vi "Initialize.vi"(8 "error in (no error)":errorcluster caption="错误输入（无错误）", 11 "虚拟 输入":refnum<class "虚拟.lvclass">) -> (0 "error out":errorcluster caption="错误输出", 3 "虚拟 输出":refnum<class "虚拟.lvclass">)   [LabVIEW 2020, in "虚拟.lvclass"]
uses:
  D:/Workspace/LabVIEW/MemristorCharacterization/Lib/2601B/2601B.lvclass
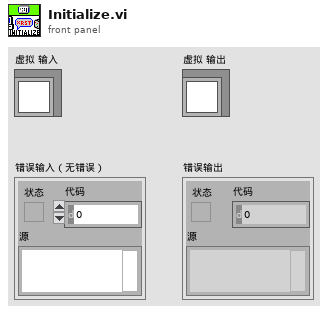
[diagram p1: front panel]
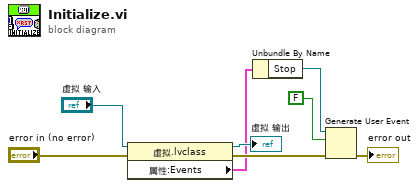
[diagram p0: block diagram]
diagram:
  n1 = property class="虚拟.lvclass"(reference="虚拟 输入", error in="error in (no error)") -> (reference out=→"虚拟 输出":refnum<class "虚拟.lvclass">, error out=w6:errorcluster, "属性:Events"=w3:cluster{"Stop":refnum<user-event>})
  n2 = Unbundle By Name(w3) -> ("Stop"=w2:refnum<user-event>)
  n3 = Generate User Event(user event=w2, event data cluster=FALSE ("事件数据"), error in=w6) -> (error out=→"error out":errorcluster)  [unwired: 1 in, 1 out]
